vi "Generador.vi"() -> (0 "Signal":dbl[](array[numeric]))   [LabVIEW 2020]
uses:
  <vilib>/Analysis/NI_AALBase.lvlib
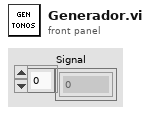
[diagram p1: front panel]
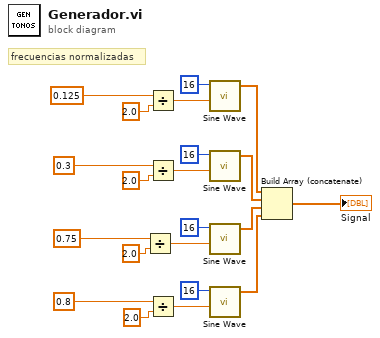
[diagram p0: block diagram]
diagram:
  # "frecuencias normalizadas"
  n1 = Divide(x=0.75 ("frequency 4"), y=2.0) -> (x/y=w20:dbl)
  n2 = Divide(x=0.125 ("frequency"), y=2.0) -> (x/y=w11:dbl)
  n3 = Divide(x=0.3 ("frequency 2"), y=2.0) -> (x/y=w19:dbl)
  n4 = Divide(x=0.8 ("frequency 3"), y=2.0) -> (x/y=w21:dbl)
  n5 = call <vilib>:"Sine Wave.vi"("samples"=16, "frequency"=w11) -> ("sine wave"=w5:dbl[])  [unwired: 3 in, 2 out]
  n6 = call <vilib>:"Sine Wave.vi"("samples"=16, "frequency"=w19) -> ("sine wave"=w6:dbl[])  [unwired: 3 in, 2 out]
  n7 = call <vilib>:"Sine Wave.vi"("samples"=16, "frequency"=w20) -> ("sine wave"=w7:dbl[])  [unwired: 3 in, 2 out]
  n8 = call <vilib>:"Sine Wave.vi"("samples"=16, "frequency"=w21) -> ("sine wave"=w8:dbl[])  [unwired: 3 in, 2 out]
  n9 = Build Array (concatenate)(w5, w6, w7, w8) -> (→"Signal":dbl[])
